vi "RampToZero.vi"(8 "error in (no error)":errorcluster, 11 "PS Driver AMI4xx.lvlib:PS Driver AMI4xx.lvclass in":refnum<class "PS Driver AMI4xx.lvclass">) -> (0 "error out":errorcluster, 3 "PS Driver AMI4xx.lvlib:PS Driver AMI4xx.lvclass out":refnum<class "PS Driver AMI4xx.lvclass">)   [LabVIEW 2020, in "PS Driver.lvlib" / "PS Driver AMI4xx.lvclass"]
uses:
  PS Driver AMI4xx.lvclass
  PS Driver with Persistence.lvclass
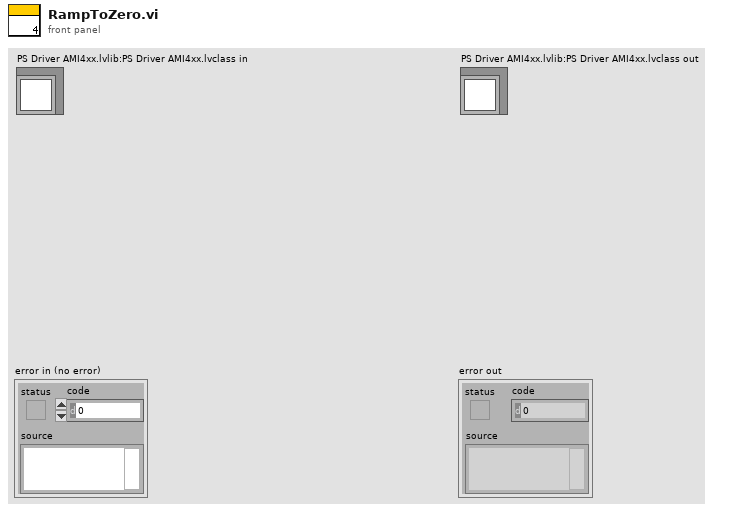
[diagram p1: front panel]
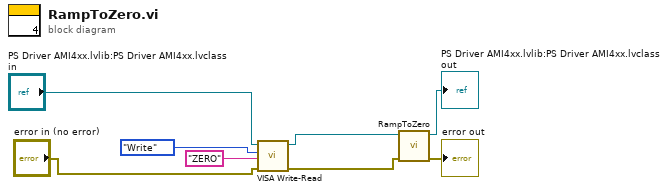
[diagram p0: block diagram]
diagram:
  n1 = call "VISA Write-Read.vi"("error in (no error)"="error in (no error)", "Command String"="ZERO", "Action"=enum16{"Write", "Read", "Write & Read"}."Write", "PS Driver.lvlib:PS Driver AMI4xx.lvclass"="PS Driver AMI4xx.lvlib:PS Driver AMI4xx.lvclass in") -> ("error out"=w1:errorcluster, "PS Driver.lvlib:PS Driver AMI4xx.lvclass out"=w2:refnum<class "PS Driver AMI4xx.lvclass">)  [unwired: 4 in, 2 out]
  n2 = call-parent "RampToZero.vi"("error in (no error)"=w1, "PS Driver.lvlib:PS Driver.lvclass in"=w2) -> ("error out"=→"error out":errorcluster, "PS Driver.lvlib:PS Driver.lvclass out"=→"PS Driver AMI4xx.lvlib:PS Driver AMI4xx.lvclass out":refnum<class "PS Driver AMI4xx.lvclass">)  [unwired: 8 in]
